vi "pump.vi"(7 "LabVIEW Web Service Request":refnum<class "Web Request.lvclass">) -> (3 "Data":dbl format="%#_13g")   [LabVIEW 2019]
uses:
  <vilib>/wsapi/Web Request.lvclass
panel:
  # "Use the Web Service Request input terminal to call the VIs on the Web Services palette. Do not remove it from the connector pane unless you don't need access to the palette."
  # "Each additional control wired to the connector pane will be available as an input in the URL. To include an indicator in terminal-mode output (the default setting), it must also be wired to the connector pane."
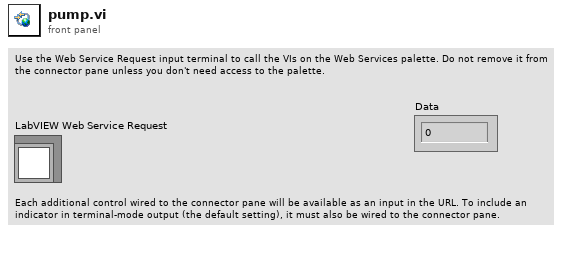
[diagram p1: front panel]
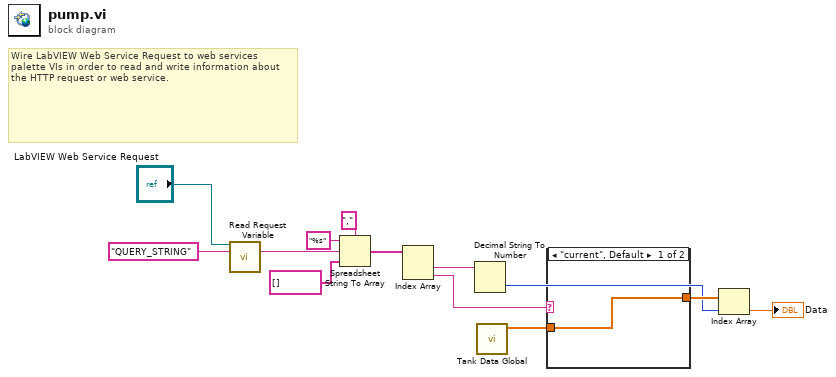
[diagram p0: block diagram]
diagram:
  # "Wire LabVIEW Web Service Request to web services palette VIs in order to read and write information about the HTTP request or web service."
  n1 = call <vilib>:"Read Request Variable.vi"("LabVIEW Web Service Request"="LabVIEW Web Service Request", "variable name"="QUERY_STRING" ("key")) -> ("value"=w12:string)  [unwired: 11 in, 2 out]
  n2 = Spreadsheet String To Array(delimiter (Tab)=",", format string="%s", spreadsheet string=w12, array type (2D Dbl)=string[] []) -> (array=w8:string[])
  n3 = Index Array(array=w8) -> (element #1=w7:string, element #2=w6:string)  [unwired: 2 in]
  n4 = Decimal String To Number(string=w7) -> (number=w3:i32)  [unwired: 2 in, 1 out]
  n5 = call "Tank Data Global.vi"() -> ("Tank Data OUT"=w5:dbl[])  [unwired: 11 in]
  n6 = case shown="\"current\", Default" w6 {
    tunnel: w5 -> [w14 w15]
    tunnel: [w14 w15] -> w4
    frame "current", Default {
    }
    frame "speed" {
    }
  }
  n7 = Index Array(array=w4, index=w3) -> (element=→"Data":dbl)
